vi "single com port capture vi.vi"(10 "unique queue name":string, 11 "Reference to control Array":refnum<vi>[](array[refnum])) -> (0 "error out":errorcluster, 3 "Reference to control Array Out":refnum<vi>[](array[refnum]))   [LabVIEW 2011]
uses:
  COM Port Control.ctl
  <vilib>/Instr/_visa.llb/VISA Configure Serial Port (Instr).vi
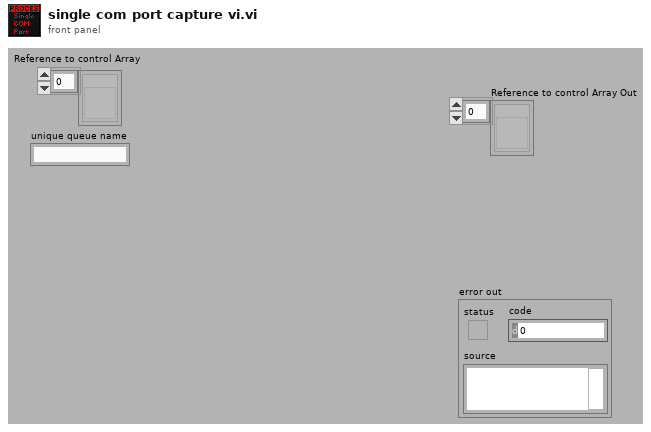
[diagram p1: front panel]
types:
  T1 = typedef "COM Port Control.ctl" = cluster{"flow control":u16, "COM Port":refnum<visa-resource-name>, "parity":enum16{"None", "Odd", "Even", "Mark", "Space"}, "data bits":u16, "baud rate":u32}
  T2 = cluster{"Number of hours To Collect before starting new file ":u16, "Base File Path":path, "Update setup":bool, "Shutdown software":bool, "Time between samples (seconds)":u32}
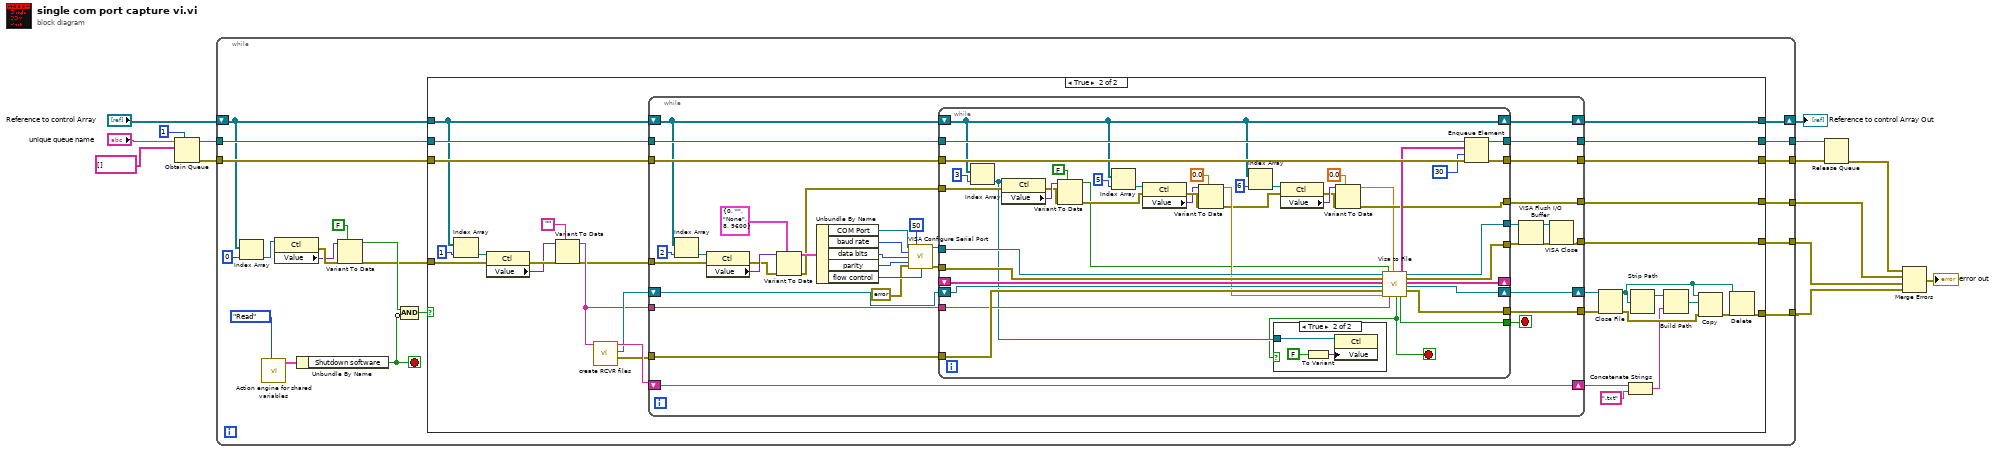
[diagram p0: block diagram]
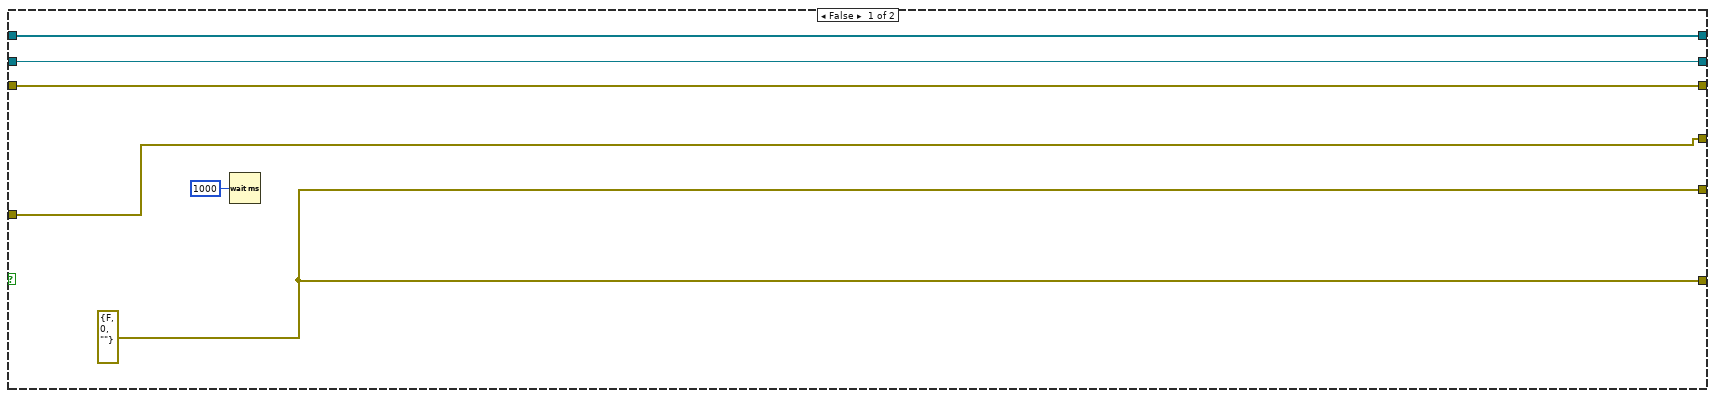
[diagram p2: hidden frame]
diagram:
  n1 = Obtain Queue(max queue size (-1, unlimited)=1, name (unnamed)="unique queue name", element data type=string[] [] ("Last 10 RCVR 1")) -> (queue out=w8:refnum<queue>, error out=w7:errorcluster)  [unwired: 2 in, 1 out]
  n2 = while {
    tunnel: [w33] -> w14
    tunnel: [w34] -> w13
    tunnel: [w22] -> w12
    tunnel: w8 -> [w21]
    tunnel: w7 -> [w20]
    tunnel: [w19] -> w5
    tunnel: [w18] -> w4
    shift-right: [w17] -> w1
    shift-left: "Reference to control Array" -> [w16]
    stop <- w29 stop-if-true
    n3 = Index Array(array=w16, index=0) -> (element=w15:refnum<vi>)
    n4 = call "Action engine for shared variables.vi"("read/write"=enum16{"Read", "Write"}."Read") -> ("func global variables read"=w30:T2)  [unwired: 9 in, 1 out]
    n5 = property class="Ctl"(reference=w15) -> (error out=w27:errorcluster, "Value"=w25:variant)  [unwired: 1 in, 1 out]
    n6 = Unbundle By Name(w30) -> ("Shutdown software"=w29:bool)
    n7 = Variant To Data(error in=w27, type=FALSE, Variant=w25) -> (data=w24:bool, error out=w23:errorcluster)
    n8 = Compound Arithmetic op=AND(w24, invert w29) -> (w32:bool)
    n9 = case shown="True" w32 {
      tunnel: [w39 w68] -> w34
      tunnel: [w39 w62] -> w33
      tunnel: w23 -> [w38 w49]
      tunnel: [w38 w47] -> w22
      tunnel: w21 -> [w37 w46]
      tunnel: w20 -> [w36 w45]
      tunnel: [w37 w44] -> w19
      tunnel: [w36 w43] -> w18
      tunnel: w16 -> [w35 w41]
      tunnel: [w35 w42] -> w17
      frame False {
        w39 = errorcluster {"status"=FALSE, "code"=0, "source"=""} ("error in (no error)")
        n10 = Wait (ms)(milliseconds to wait=u32 1000) -> ()  [unwired: 1 out]
      }
      frame True {
        n11 = Index Array(array=w41, index=1) -> (element=w54:refnum<vi>)
        n12 = property class="Ctl"(reference=w54, error in=w49) -> (error out=w53:errorcluster, "Value"=w52:variant)  [unwired: 1 out]
        n13 = Variant To Data(error in=w53, type="", Variant=w52) -> (data=w50:string, error out=w48:errorcluster)
        n14 = call "create RCVR files.vi"("Name of RCVR 1"=w50) -> ("error out"=w56:errorcluster, "refnum out"=w57:refnum<file>, "Name of file out"=w58:string)  [unwired: 8 in]
        n15 = while {
          tunnel: w56 -> [w105]
          tunnel: [w89] -> w69
          tunnel: [w95] -> w68
          shift-right: [w87] -> w61
          shift-left: w58 -> [w87]
          tunnel: w50 -> [w86]
          tunnel: w48 -> [w79]
          tunnel: [w77] -> w47
          tunnel: w46 -> [w76]
          tunnel: w45 -> [w75]
          tunnel: [w74] -> w44
          tunnel: [w73] -> w43
          shift-right: [w72] -> w42
          shift-left: w41 -> [w71]
          shift-right: [w97] -> w70
          shift-left: w57 -> [w106]
          stop <- w88 stop-if-true
          n16 = Index Array(array=w71, index=2) -> (element=w83:refnum<vi>)
          n17 = property class="Ctl"(reference=w83, error in=w79) -> (error out=w84:errorcluster, "Value"=w85:variant)  [unwired: 1 out]
          n18 = Variant To Data(error in=w84, type=T1 {"flow control"=0, "COM Port"="", "parity"=enum."None", "data bits"=8, "baud rate"=9600} ("COM Port 1"), Variant=w85) -> (data=w81:T1, error out=w78:errorcluster)
          n19 = Unbundle By Name(w81) -> ("COM Port"=w102:refnum<visa-resource-name>, "baud rate"=w101:u32, "data bits"=w100:u16, "parity"=w99:enum16{"None", "Odd", "Even", "Mark", "Space"}, "flow control"=w98:u16)
          n20 = call-poly "VISA Configure Serial Port"("VISA resource name"=w102, "timeout (10sec)"=u32 50, "baud rate (9600)"=w101, "data bits (8)"=w100, "parity (0:none)"=w99, "error in (no error)"=errorcluster {"status"=FALSE, "code"=0, "source"=""}, "flow control (0:none)"=w98) -> ("VISA resource name out"=w104:refnum<visa-resource-name>, "error out"=w103:errorcluster)  [unwired: 7 in]
          n21 = while {
            tunnel: [w144] -> w91
            tunnel: w105 -> [w138]
            tunnel: w104 -> [w148]
            tunnel: [w141] -> w89
            tunnel: [w140] -> w88
            shift-right: [w145] -> _
            shift-left: _ -> [w146]
            tunnel: w103 -> [w147]
            tunnel: [w143] -> w92
            tunnel: w86 -> [w137]
            tunnel: w78 -> [w133]
            tunnel: [w108] -> w77
            tunnel: w76 -> [w131]
            tunnel: w75 -> [w130]
            tunnel: [w127] -> w74
            tunnel: [w126] -> w73
            shift-right: [w110] -> w72
            shift-left: w71 -> [w110]
            shift-right: [w142] -> w97
            shift-left: w106 -> [w139]
            stop <- w116 stop-if-true
            n22 = Index Array(array=w110, index=3) -> (element=w117:refnum<vi>)
            n23 = property class="Ctl"(reference=w117, error in=w133) -> (error out=w132:errorcluster, "Value"=w135:variant)  [unwired: 1 out]
            n24 = Variant To Data(error in=w132, type=FALSE, Variant=w135) -> (data=w118:bool, error out=w121:errorcluster)
            n25 = Index Array(array=w110, index=5) -> (element=w123:refnum<vi>)
            n26 = property class="Ctl"(reference=w123, error in=w121) -> (error out=w125:errorcluster, "Value"=w124:variant)  [unwired: 1 out]
            n27 = Variant To Data(error in=w125, type=0.0 ("Antenna offset"), Variant=w124) -> (data=w119:dbl, error out=w111:errorcluster)
            n28 = Index Array(array=w110, index=6) -> (element=w114:refnum<vi>)
            n29 = property class="Ctl"(reference=w114, error in=w111) -> (error out=w112:errorcluster, "Value"=w113:variant)  [unwired: 1 out]
            n30 = Variant To Data(error in=w112, type=0.0 ("Antenna offset"), Variant=w113) -> (data=w107:dbl, error out=w108:errorcluster)
            n31 = call "Visa to File.vi"("VISA resource name in"=w148, "Visa Error"=w147, "Array in from shift reg"=w146, "File data refnum"=w139, "File handle Error"=w138, "Antenna offset"=w119, "UPDT COM switch"=w118, "Name of RCVR 1"=w137, "Grennich Offset"=w107) -> ("End Visa Loop"=w116:bool, "Last 10 RCVR 1"=w128:string[], "End File Loop"=w140:bool, "VISA resource name out"=w144:refnum<visa-resource-name>, "Visa error out"=w143:errorcluster, "Array out to shift reg"=w145:string[], "File data refnum out"=w142:refnum<file>, "File Error out"=w141:errorcluster)  [unwired: 3 in]
            n32 = case shown="True" w116 {
              tunnel: w117 -> [_ w151]
              frame False {
              }
              frame True {
                n33 = To Variant(anything=FALSE) -> (Variant=w150:variant)
                n34 = property class="Ctl"(reference=w151, "Value"=w150) -> ()  [unwired: 1 in, 2 out]
              }
            }
            n35 = Enqueue Element(queue=w131, element=w128, timeout in ms (-1)=30, error in (no error)=w130) -> (queue out=w127:refnum<queue>, error out=w126:errorcluster)  [unwired: 1 out]
          }
          n36 = VISA Flush I/O Buffer(VISA resource name=w91, error in (no error)=w92) -> (VISA resource name out=w94:refnum<visa-resource-name>, error out=w93:errorcluster)  [unwired: 1 in]
          n37 = VISA Close(VISA resource name=w94, error in (no error)=w93) -> (error out=w95:errorcluster)
        }
        n38 = Close File(refnum=w70, error in=w69) -> (path=w63:path, error out=w64:errorcluster)
        n39 = Concatenate Strings(w61, ".txt" ("string")) -> (w59:string)
        n40 = Strip Path(path=w63) -> (stripped path=w66:path)  [unwired: 1 out]
        n41 = Build Path(base path=w66, name or relative path=w59) -> (appended path=w67:path)
        n42 = Copy(8:w64, 10:w67, 11:w63) -> (0:w65:errorcluster)  [unwired: 2 in, 2 out]
        n43 = Delete(path (use dialog)=w63, error in=w65) -> (error out=w62:errorcluster)  [unwired: 3 in, 2 out]
      }
    }
  }
  "Reference to control Array Out" <- w1
  n44 = Release Queue(queue=w5, error in (no error)=w4) -> (error out=w3:errorcluster)  [unwired: 1 in, 2 out]
  n45 = Merge Errors(w3, w12, w13, w14) -> (→"error out":errorcluster)
